vi "RunAllTests.vi"() -> ()   [LabVIEW 2019]
panel:
  out "Trajectory":bool
  out "Path":bool
  out "Path Constraints":bool
  out "Constraints Zone":bool
  out "All Tests Finished":bool
  out "Geometry Util":bool
  # "FORMAL PathPlannerLib LabVIEW TEST PROCEDURE"
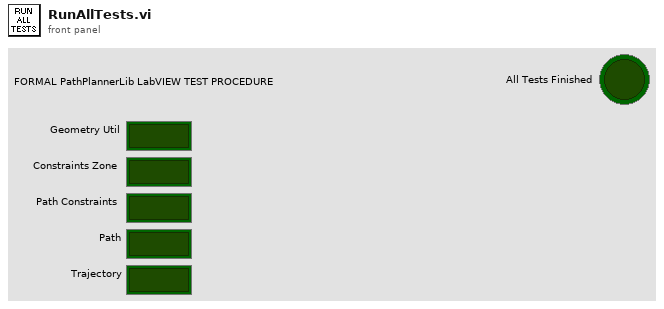
[diagram p1: front panel]
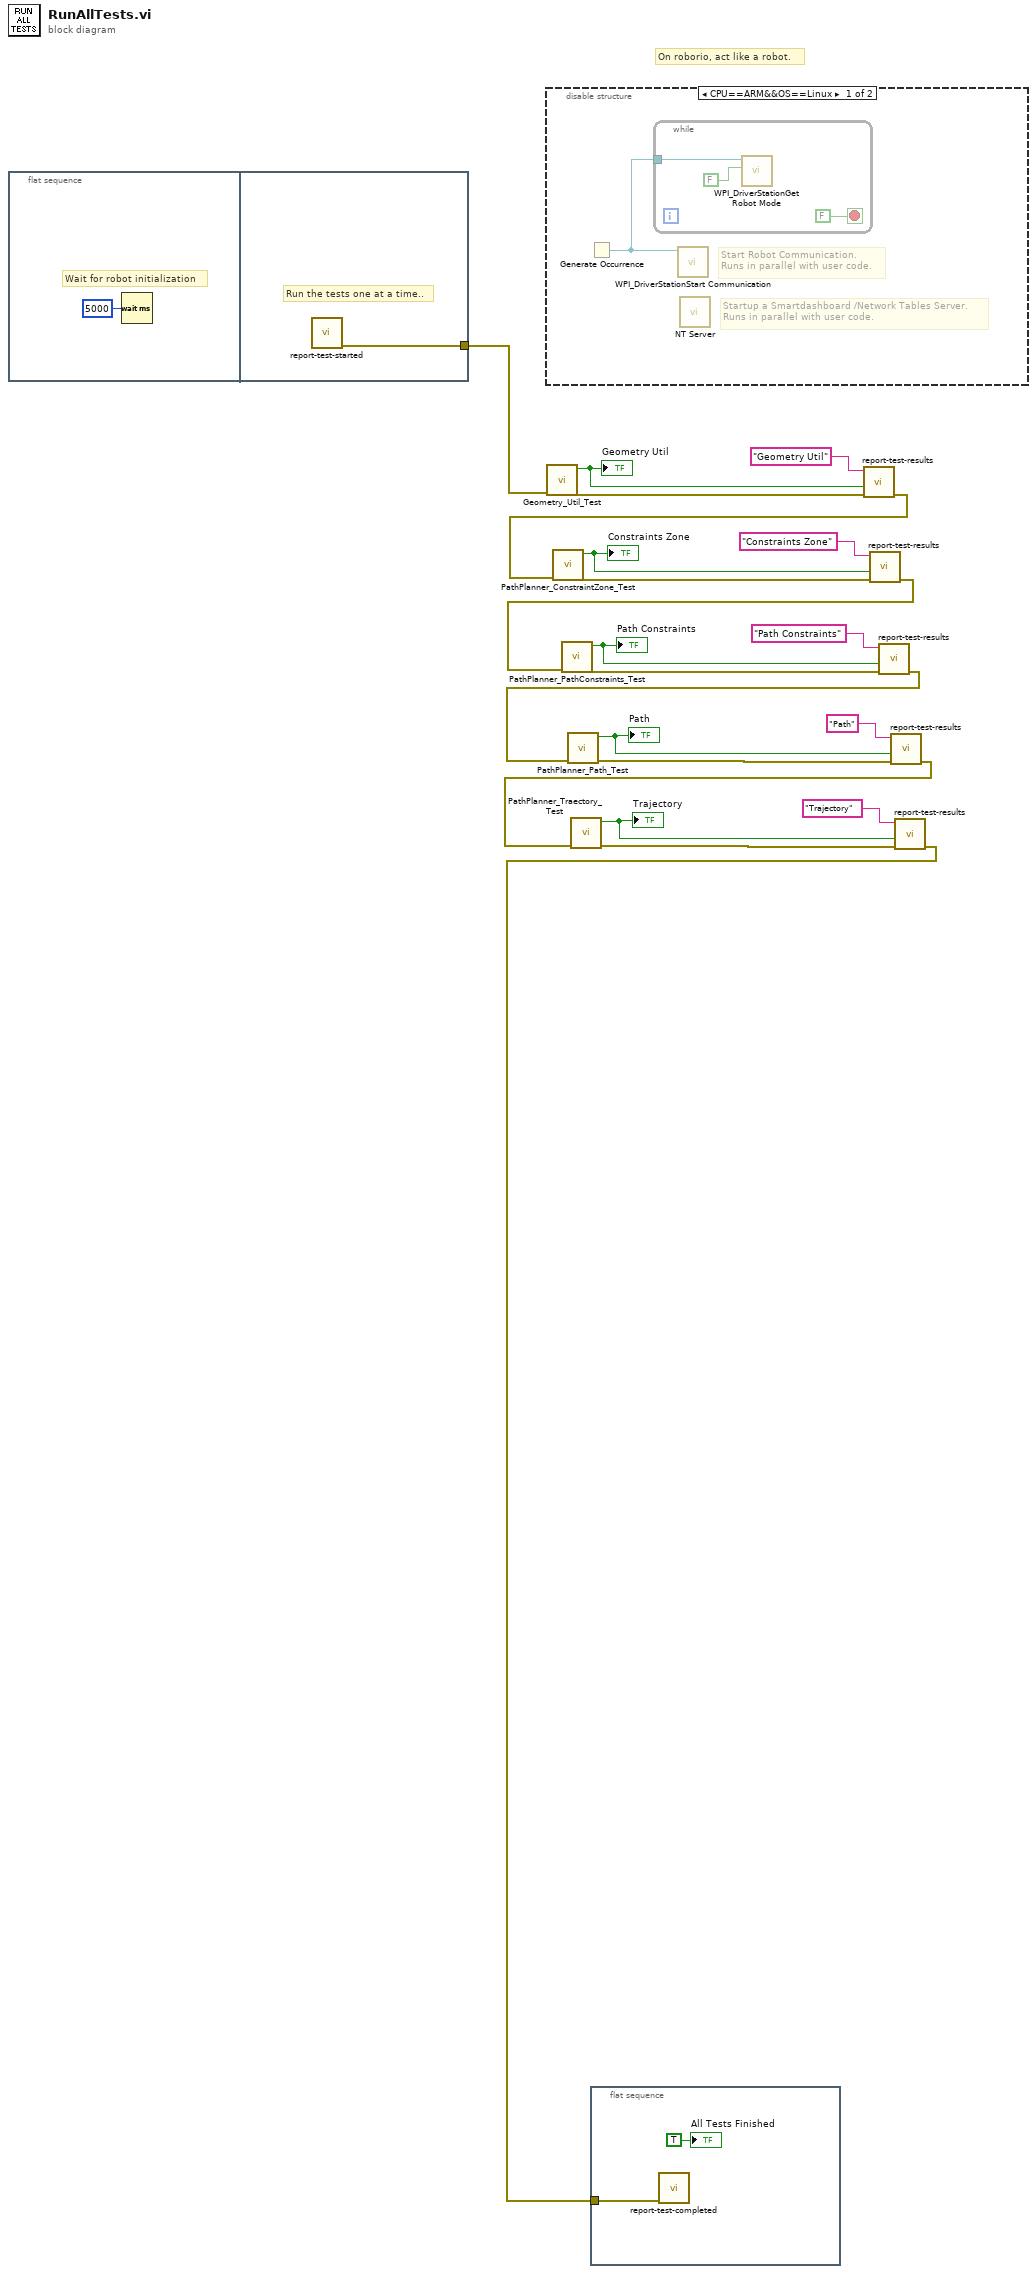
[diagram p0: block diagram]
diagram:
  # "On roborio, act like a robot."
  n1 = flat-sequence {
    tunnel: [w23] -> w18
    frame #0 {
      # "Wait for robot initialization"
      n2 = Wait (ms)(milliseconds to wait=u32 5000) -> ()  [unwired: 1 out]
    }
    frame #1 {
      # "Run the tests one at a time.."
      n3 = call "report-test-started.vi"() -> ("error out"=w23:errorcluster)  [unwired: 11 in]
    }
  }
  n4 = disable-structure shown="CPU==ARM&&OS==Linux" {
    frame condition #0 {
      # "Startup a Smartdashboard /Network Tables Server.\nRuns in parallel with user code."
      # "Start Robot Communication.\nRuns in parallel with user code."
      n5 = Generate Occurrence() -> (w24:refnum<k4>)
      n6 = while {
        tunnel: w24 -> [w27]
        stop <- FALSE stop-if-true
        n7 = call <vilib>:"WPI_DriverStationGet Robot Mode.vi"("Finish"=FALSE, "DS Occurrence"=w27) -> ()  [unwired: 10 out]
      }
      n8 = call <vilib>:"WPI_DriverStationStart Communication.vi"("occurrence"=w24) -> ()  [unwired: 2 in, 9 out]
      n9 = call <vilib>:"NT Server.vi"() -> ()  [unwired: 11 in, 1 out]
    }
    frame condition #1 (active) {
    }
  }
  n10 = call "Geometry_Util_Test.vi"("error in (no error)"=w18) -> ("error out"=w19:errorcluster, "All Passed"=w21:bool)  [unwired: 9 in]
  "Geometry Util" <- w21
  n11 = flat-sequence {
    tunnel: w4 -> [w28]
    frame #0 {
      n12 = call "report-test-completed.vi"("error in (no error)"=w28) -> ()  [unwired: 10 in, 1 out]
      "All Tests Finished" <- TRUE ("All Tests Finished")
    }
  }
  n13 = call "report-test-results.vi"("error in (no error)"=w19, "TestPassed"=w21, "Test Name"="Geometry Util") -> ("error out"=w15:errorcluster)  [unwired: 8 in]
  n14 = call "PathPlanner_ConstraintZone_Test.vi"("error in (no error)"=w15) -> ("error out"=w16:errorcluster, "All Passed"=w14:bool)  [unwired: 9 in]
  "Constraints Zone" <- w14
  n15 = call "report-test-results.vi"("error in (no error)"=w16, "TestPassed"=w14, "Test Name"="Constraints Zone") -> ("error out"=w10:errorcluster)  [unwired: 8 in]
  n16 = call "PathPlanner_PathConstraints_Test.vi"("error in (no error)"=w10) -> ("error out"=w12:errorcluster, "All Passed"=w11:bool)  [unwired: 9 in]
  "Path Constraints" <- w11
  n17 = call "report-test-results.vi"("error in (no error)"=w12, "TestPassed"=w11, "Test Name"="Path Constraints") -> ("error out"=w8:errorcluster)  [unwired: 8 in]
  n18 = call "PathPlanner_Path_Test.vi"("error in (no error)"=w8) -> ("error out"=w7:errorcluster, "All Passed"=w6:bool)  [unwired: 9 in]
  "Path" <- w6
  n19 = call "report-test-results.vi"("error in (no error)"=w7, "TestPassed"=w6, "Test Name"="Path") -> ("error out"=w3:errorcluster)  [unwired: 8 in]
  n20 = call "PathPlanner_Traectory_Test.vi"("error in (no error)"=w3) -> ("error out"=w2:errorcluster, "All Passed"=w1:bool)  [unwired: 9 in]
  "Trajectory" <- w1
  n21 = call "report-test-results.vi"("error in (no error)"=w2, "TestPassed"=w1, "Test Name"="Trajectory") -> ("error out"=w4:errorcluster)  [unwired: 8 in]
